vi "TFSA - TF and Coherence V2.vi"(0 "wForms IN":waveform(dbl)[](array[waveform]), 5 "error in (no error)":errorcluster, 6 "Spectral Function Parameters":T1={"Frequency resolution (Hz)"=1.0, "Overlap"=0.0, "Window"=0} {"Window" items=["Rectangle"=0, "Hanning"=1, "Hamming"=2, "Blackman-Harris"=3, "Exact Blackman"=4, "Blackman"=5, "Flat Top"=6, "4 Term B-Harris "=7, "7 Term B-Harris"=8, "Low Sidelobe"=9, "Blackman Nuttall"=11, "Triangle"=30, "Bartlett-Hanning"=31, "Bohman"=32, "Parzen"=33, "Welch"=34, "Kaiser"=60, "Dolph-Chebyshev"=61, "Gaussian"=62]}, 7 "Reference Indexes":i32[](array[numeric]), 9 "Response Indexes":i32[](array[numeric])) -> (14 "TF OUT":waveform(cdb)[](array[waveform]), 15 "Coherence":waveform(dbl)[](array[waveform]), 16 "Nb Averages":i32[](array[numeric]), 17 "Nb TF":i32, 19 "error out":errorcluster)   [LabVIEW 2020, in "GSwFormDSP.lvclass"]
uses:
  GSwFormDSP.lvclass
  Spectral Parameters.ctl
  <vilib>/Analysis/4window.llb/windowTd.ctl
  Attribute List.ctl
  <vilib>/Analysis/0measdsp.llb/Scaled Time Domain Window (DBL).vi
  <vilib>/Analysis/NI_AALPro.lvlib
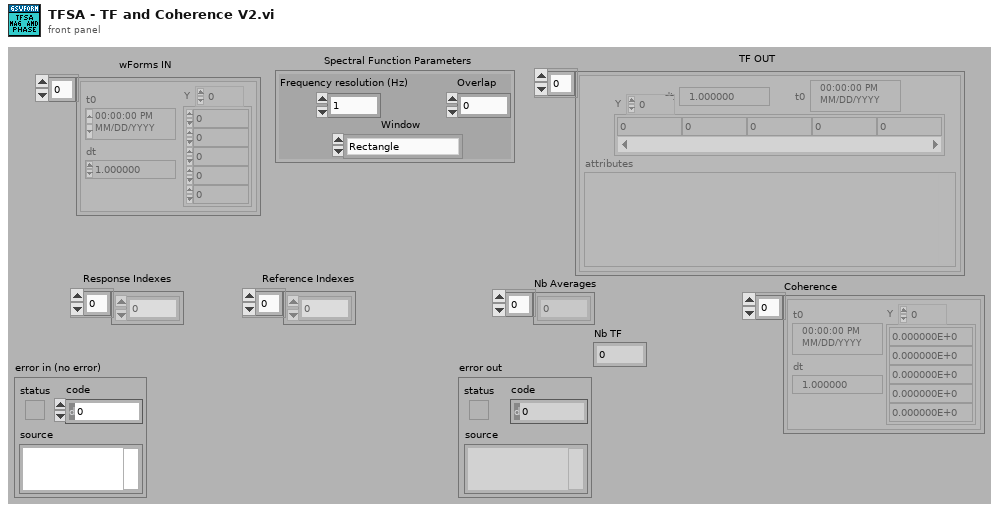
[diagram p1: front panel]
types:
  T1 = typedef "GSwFormDSP.lvclass/Spectral Parameters.ctl" = cluster{"Frequency resolution (Hz)":dbl, "Overlap":dbl, "Window":T2}
  T2 = typedef "NI_AALPro.lvlib/windowTd.ctl" = u32
  T3 = typedef "GSwFormDSP.lvclass/Attribute List.ctl" = string
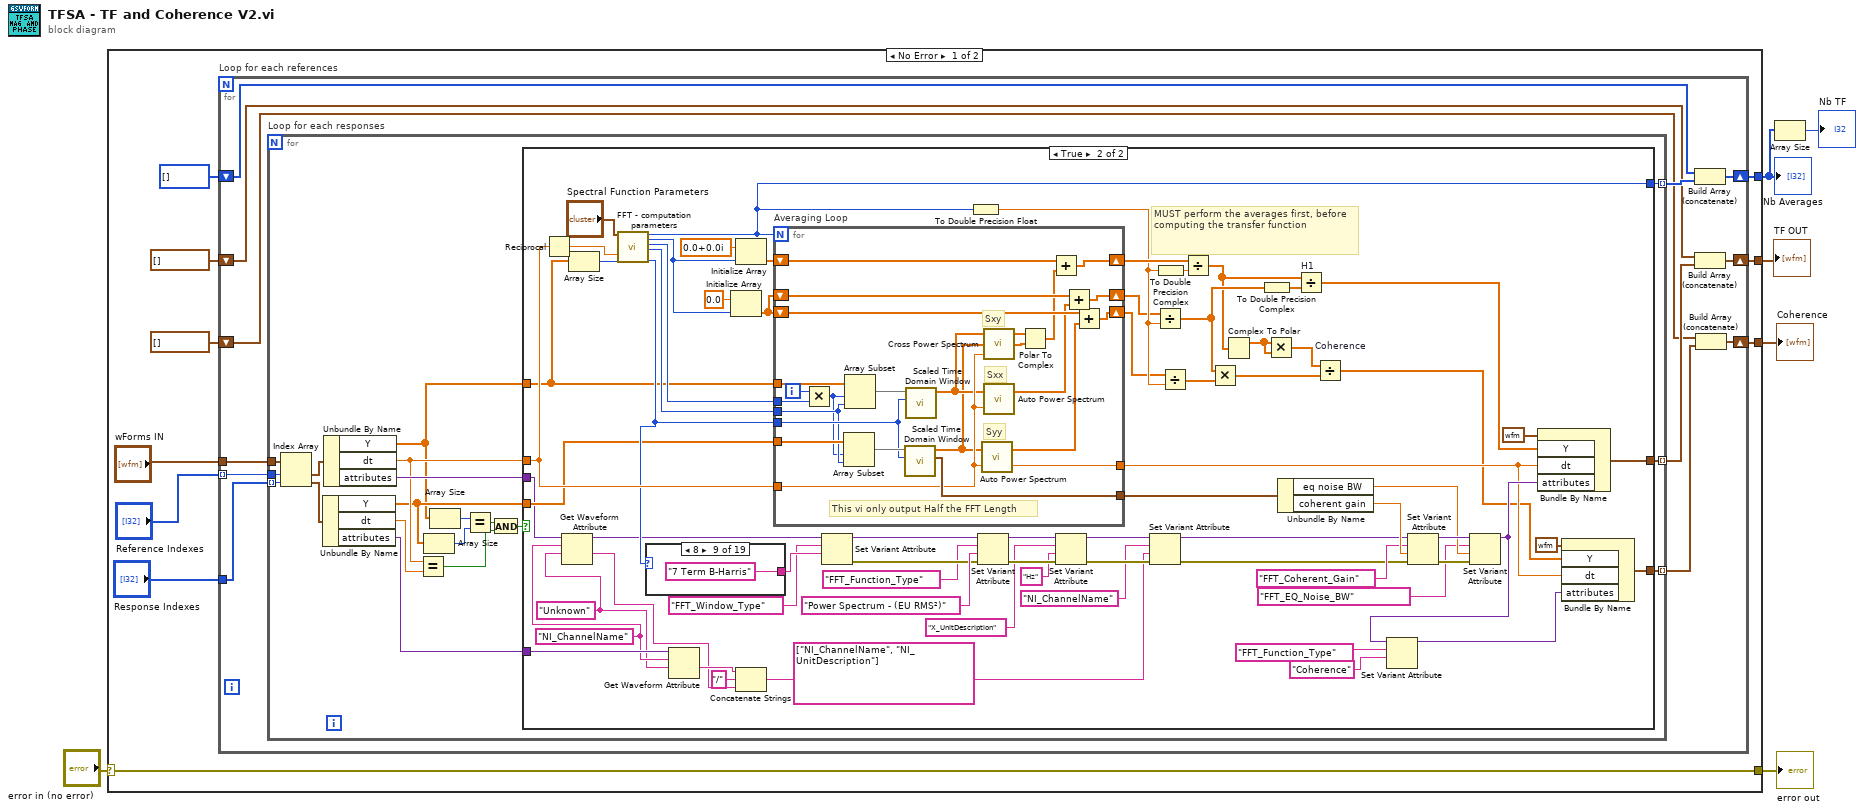
[diagram p0: block diagram]
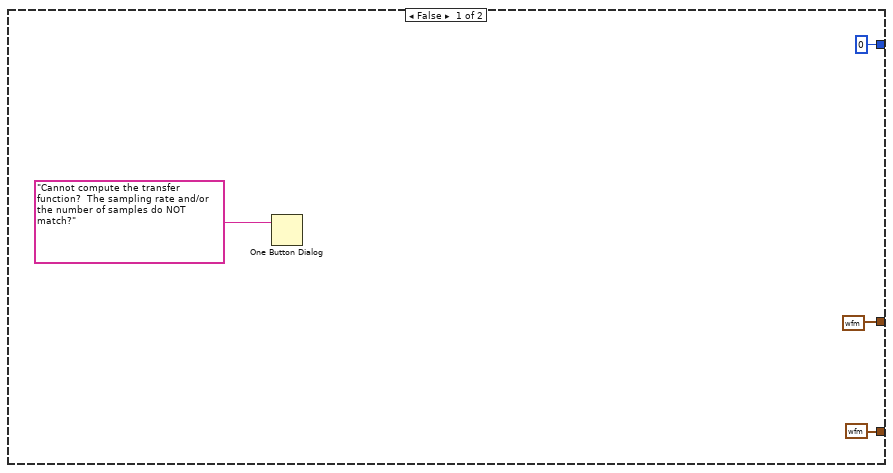
[diagram p2: hidden frame]
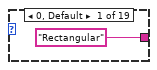
[diagram p3: hidden frame]
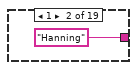
[diagram p4: hidden frame]
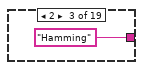
[diagram p5: hidden frame]
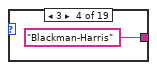
[diagram p6: hidden frame]
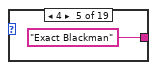
[diagram p7: hidden frame]
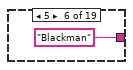
[diagram p8: hidden frame]
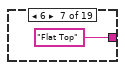
[diagram p9: hidden frame]
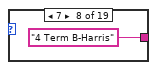
[diagram p10: hidden frame]
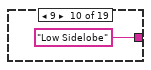
[diagram p11: hidden frame]
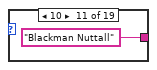
[diagram p12: hidden frame]
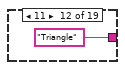
[diagram p13: hidden frame]
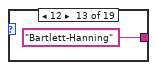
[diagram p14: hidden frame]
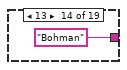
[diagram p15: hidden frame]
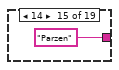
[diagram p16: hidden frame]
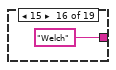
[diagram p17: hidden frame]
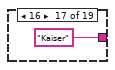
[diagram p18: hidden frame]
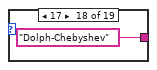
[diagram p19: hidden frame]
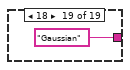
[diagram p20: hidden frame]
diagram:
  n1 = case shown="No Error" "error in (no error)" {
    selector: "error in (no error)" -> [w13 w168]
    tunnel: [w13 w168] -> w5
    tunnel: [w9 waveform(cdb)[] [] ("wForms IN")] -> w4
    tunnel: [w8 i32[] []] -> w2
    tunnel: [w7 waveform(dbl)[] []] -> w3
    frame No Error {
      n2 = for "Loop for each references" {
        tunnel: "wForms IN" -> [w28]
        tunnel: "Reference Indexes" -> [w27] mode=indexing
        tunnel: "Response Indexes" -> [w26]
        shift-right: [w24] -> w8
        shift-left: i32[] [] -> [w23]
        shift-right: [w22] -> w9
        shift-left: waveform(cdb)[] [] -> [w20]
        shift-right: [w19] -> w7
        shift-left: waveform(dbl)[] [] -> [w17]
        n3 = for "Loop for each responses" {
          tunnel: [w47] -> w21 mode=indexing
          tunnel: w28 -> [w44]
          tunnel: [w45] -> w25 mode=indexing
          tunnel: w27 -> [w43]
          tunnel: w26 -> [w42] mode=indexing
          tunnel: [w29] -> w18 mode=indexing
          n4 = Index Array(array=w44, index #1=w43, index #2=w42) -> (element #1=w41:waveform(dbl), element #2=w40:waveform(dbl))
          n5 = Unbundle By Name(w40) -> ("Y"=w37:dbl[], "dt"=w38:dbl, "attributes"=w30:variant)
          n6 = Unbundle By Name(w41) -> ("Y"=w36:dbl[], "dt"=w39:dbl, "attributes"=w46:variant)
          n7 = Equal?(x=w39, y=w38) -> (x = y?=w32:bool)
          n8 = Array Size(array=w37) -> (size(s)=w34:i32)
          n9 = Array Size(array=w36) -> (size(s)=w35:i32)
          n10 = Equal?(x=w35, y=w34) -> (x = y?=w33:bool)
          n11 = And(x=w33, y=w32) -> (x .and. y?=w31:bool)
          n12 = case shown="True" w31 {
            tunnel: [waveform(cdb) {"t0"=timestamp(0 s since 1904-01-01), "dt"=1.0, "Y"=[]} ("Waveform") w120] -> w47
            tunnel: w39 -> [_ w115]
            tunnel: w46 -> [_ w90]
            tunnel: w36 -> [_ w101]
            tunnel: [0 ("Nb Averages") w96] -> w45
            tunnel: w37 -> [_ w98]
            tunnel: w30 -> [_ w88]
            tunnel: [waveform(dbl) {"t0"=timestamp(0 s since 1904-01-01), "dt"=1.0, "Y"=[]} ("Waveform") w70] -> w29
            frame False {
              n13 = One Button Dialog(message="Cannot compute the transfer function?  The sampling rate and/or the number of samples do NOT match?") -> ()  [unwired: 1 in, 1 out]
            }
            frame True {
              (unwired) T3[] ["NI_ChannelName", "NI_UnitDescription"] ("Attribute List")
              w86 = "Unknown" ("Abscissa.Unit (X)")
              w87 = T3 "NI_ChannelName" ("wForm Attributes")
              # "MUST perform the averages first, before computing the transfer function"
              n14 = Reciprocal(x=w115) -> (1/x=w116:dbl)
              n15 = Get Waveform Attribute(5:w86, 6:w87, 7:w90) -> (1:w83:string, 3:w89:variant)  [unwired: 1 in, 2 out]
              n16 = Array Size(array=w101) -> (size(s)=w117:i32)
              n17 = call "FFT - computation parameters.vi"("Spectral Function Parameters"="Spectral Function Parameters", "Fs"=w116, "Time vector length (samples)"=w117) -> ("Nb Averages"=w96:i32, "FFT Length/2"=w55:i32, "FFT Length - Overlap"=w118:i32, "FFT Length"=w103:i32, "window"=w102:T2)  [unwired: 11 in, 1 out]
              n18 = case shown="8" w102 {
                tunnel: ["Rectangular" ("Abscissa.Unit (X)") "Hanning" ("Abscissa.Unit (X)") "Hamming" ("Abscissa.Unit (X)") "Blackman-Harris" ("Abscissa.Unit (X)") "Exact Blackman" ("Abscissa.Unit (X)") "Blackman" ("Abscissa.Unit (X)") "Flat Top" ("Abscissa.Unit (X)") "4 Term B-Harris" ("Abscissa.Unit (X)") "7 Term B-Harris" ("Abscissa.Unit (X)") "Low Sidelobe" ("Abscissa.Unit (X)") "Blackman Nuttall" ("Abscissa.Unit (X)") "Triangle" ("Abscissa.Unit (X)") "Bartlett-Hanning" ("Abscissa.Unit (X)") "Bohman" ("Abscissa.Unit (X)") "Parzen" ("Abscissa.Unit (X)") "Welch" ("Abscissa.Unit (X)") "Kaiser" ("Abscissa.Unit (X)") "Dolph-Chebyshev" ("Abscissa.Unit (X)") "Gaussian" ("Abscissa.Unit (X)")] -> w114
                frame 0, Default {
                }
                frame 1 {
                }
                frame 2 {
                }
                frame 3 {
                }
                frame 4 {
                }
                frame 5 {
                }
                frame 6 {
                }
                frame 7 {
                }
                frame 8 {
                }
                frame 9 {
                }
                frame 10 {
                }
                frame 11 {
                }
                frame 12 {
                }
                frame 13 {
                }
                frame 14 {
                }
                frame 15 {
                }
                frame 16 {
                }
                frame 17 {
                }
                frame 18 {
                }
              }
              n19 = Get Waveform Attribute(5:w86, 6:w87, 7:w88) -> (1:w85:string)  [unwired: 1 in, 3 out]
              n20 = Initialize Array(0.0, w55) -> (w65:dbl[])
              n21 = Initialize Array(cdb 0.0+0.0i, w55) -> (w56:cdb[])
              n22 = Concatenate Strings(w85, "/" ("string"), w83) -> (w77:string)
              n23 = for "Averaging Loop" {
                N: w96 -> [_]
                shift-right: [w151] -> w69
                shift-left: w56 -> [w161]
                tunnel: w118 -> [w163]
                tunnel: w103 -> [w155]
                tunnel: w101 -> [w152]
                tunnel: w115 -> [w153]
                tunnel: [w160] -> w71
                tunnel: [w158] -> w119
                tunnel: w102 -> [w156]
                tunnel: w98 -> [w157]
                shift-right: [w147] -> w63
                shift-left: w65 -> [w148]
                shift-right: [w145] -> w62
                shift-left: w65 -> [w146]
                i -> [w164]
                # "Sxy"
                # "Syy"
                # "Sxx"
                # "This vi only output Half the FFT Length"
                n24 = Multiply(x=w164, y=w163) -> (x*y=w154:i32)
                n25 = Array Subset(array=w157, index=w154, length=w155) -> (w159:dbl[])
                n26 = Array Subset(array=w152, index=w154, length=w155) -> (w162:dbl[])
                n27 = call-poly <vilib>:"Scaled Time Domain Window.vi"("window"=w156, "X"=w159) -> ("window properties"=w158:cluster{"eq noise BW":dbl, "coherent gain":dbl}, "Windowed X"=w149:dbl[])  [unwired: 1 in, 7 out]
                n28 = call-poly <vilib>:"Scaled Time Domain Window.vi"("window"=w156, "X"=w162) -> ("Windowed X"=w150:dbl[])  [unwired: 1 in, 8 out]
                n29 = call <vilib>:"Auto Power Spectrum.vi"("dt"=w153, "Signal (V)"=w149) -> ("df"=w160:dbl, "Power Spectrum (V^2 rms)"=w144:dbl[])
                n30 = call <vilib>:"Cross Power Spectrum.vi"("dt"=w153, "Signal Y (V)"=w149, "Signal X (V)"=w150) -> ("Cross Power XY Spectrum Phase (radians)"=w142:dbl[], "Cross Power XY Spectrum Mag (V^2rms)"=w141:dbl[])  [unwired: 1 out]
                n31 = call <vilib>:"Auto Power Spectrum.vi"("dt"=w153, "Signal (V)"=w150) -> ("Power Spectrum (V^2 rms)"=w143:dbl[])  [unwired: 1 out]
                n32 = Polar To Complex(1:w142, 2:w141) -> (0:w140:cdb[])
                n33 = Add(x=w161, y=w140) -> (x+y=w151:cdb[])
                n34 = Add(x=w148, y=w143) -> (x+y=w147:dbl[])
                n35 = Add(x=w146, y=w144) -> (x+y=w145:dbl[])
              }
              n36 = Set Variant Attribute(Variant=w89, name=T3 "FFT_Window_Type" ("wForm Attributes"), value=w114) -> (Variant out=w113:variant, error out=w111:errorcluster)  [unwired: 1 in, 1 out]
              n37 = To Double Precision Float(number=w96) -> (double precision float=w64:dbl)
              n38 = Set Variant Attribute(Variant=w113, name=T3 "FFT_Function_Type" ("wForm Attributes"), value="Power Spectrum - (EU RMS²)" ("Ordinate.Function Description.Function Type"), error in=w111) -> (Variant out=w110:variant, error out=w109:errorcluster)  [unwired: 1 out]
              n39 = Set Variant Attribute(Variant=w110, name=T3 "X_UnitDescription" ("wForm Attributes"), value="Hz" ("Abscissa.Unit (X)"), error in=w109) -> (Variant out=w81:variant, error out=w82:errorcluster)  [unwired: 1 out]
              n40 = Set Variant Attribute(Variant=w81, name=T3 "NI_ChannelName" ("wForm Attributes"), value=w77, error in=w82) -> (Variant out=w80:variant, error out=w79:errorcluster)  [unwired: 1 out]
              n41 = Divide(x=w63, y=w64) -> (x/y=w61:dbl[])
              n42 = To Double Precision Complex(1:w64) -> (0:w54:cdb)
              n43 = Divide(x=w62, y=w64) -> (x/y=w60:dbl[])
              n44 = Divide(x=w69, y=w54) -> (x/y=w53:cdb[])
              n45 = Multiply(x=w61, y=w60) -> (x*y=w67:dbl[])
              n46 = Complex To Polar(r * e^(i*theta)=w53) -> (r=w52:dbl[])  [unwired: 1 out]
              n47 = To Double Precision Complex(1:w61) -> (0:w66:cdb[])
              n48 = Multiply(x=w52, y=w52) -> (x*y=w68:dbl[])
              n49 = Unbundle By Name(w119) -> ("eq noise BW"=w104:dbl, "coherent gain"=w107:dbl)
              n50 = Divide "H1"(x=w53, y=w66) -> (x/y=w58:cdb[])
              n51 = Divide "Coherence"(x=w68, y=w67) -> (x/y=w59:dbl[])
              n52 = Set Variant Attribute(Variant=w80, name=T3 "FFT_Coherent_Gain" ("wForm Attributes"), value=w107, error in=w79) -> (Variant out=w105:variant, error out=w106:errorcluster)  [unwired: 1 out]
              n53 = Set Variant Attribute(Variant=w105, name=T3 "FFT_EQ_Noise_BW" ("wForm Attributes"), value=w104, error in=w106) -> (Variant out=w76:variant)  [unwired: 2 out]
              n54 = Set Variant Attribute(Variant=w76, name=T3 "FFT_Function_Type" ("wForm Attributes"), value="Coherence" ("Ordinate.Function Description.Function Type")) -> (Variant out=w72:variant)  [unwired: 1 in, 2 out]
              n55 = Bundle By Name(cluster=waveform(cdb) {"t0"=timestamp(0 s since 1904-01-01), "dt"=1.0, "Y"=[]} ("Waveform"), "Y"=w58, "dt"=w71, "attributes"=w76) -> (w120:waveform(cdb))
              n56 = Bundle By Name(cluster=waveform(dbl) {"t0"=timestamp(0 s since 1904-01-01), "dt"=1.0, "Y"=[]} ("Waveform"), "Y"=w59, "dt"=w71, "attributes"=w72) -> (w70:waveform(dbl))
            }
          }
        }
        n57 = Build Array (concatenate)(w23, w25) -> (w24:i32[])
        n58 = Build Array (concatenate)(w20, w21) -> (w22:waveform(cdb)[])
        n59 = Build Array (concatenate)(w17, w18) -> (w19:waveform(dbl)[])
      }
    }
    frame Error {
    }
  }
  "error out" <- w5
  "TF OUT" <- w4
  "Nb Averages" <- w2
  "Coherence" <- w3
  n60 = Array Size(array=w2) -> (size(s)=→"Nb TF":i32)
